vi "AO Reg UI.vi"(8 "error in (no error)":errorcluster, 11 "Node Ptr":T4 format="%.0x") -> (0 "error out":errorcluster)   [LabVIEW 2015, in "Modbus Master System Explorer.lvlib"]
uses:
  Modbus Master System Explorer.lvlib
  <vilib>/NI Veristand/Custom Device API/Custom Device Item Ref.ctl
  Shared/Controls/Data Model/DataType.ctl
  SubVIs/Radix.ctl
  SubVIs/Direction.ctl
  <vilib>/NI VeriStand/Custom Device API/Custom Device API.lvlib
  Shared/Modbus Master Shared.lvlib
panel:
  in  "Direction":T1
  in  "Radix":T2
  out "Bytes":i32
  in  "Sub-Index (Bool)":u16
  in  "DataType":T3
  in  "Valid?":string
  in  "Address":u16
  in  "Header":cluster{"Section Name":string}={"Section Name"="Holding Register (Analog Out) Settings"}
  in  "Description":string
  in  "Name":string
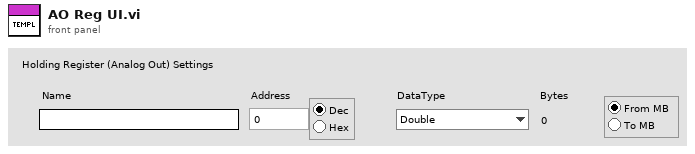
[diagram p1: front panel]
types:
  T1 = typedef "Modbus Master System Explorer.lvlib/Direction.ctl" = enum32{"Radio Selection 1", "Radio Selection 2"}
  T2 = typedef "Modbus Master System Explorer.lvlib/Radix.ctl" = enum32{"Decimal", "Hexidecimal"}
  T3 = typedef "Modbus Master Shared.lvlib/DataType.ctl" = enum16{"Double", "Single", "I64", "I32", "I16", "I8", "U64", "U32", "U16", "U8", "Boolean"}
  T4 = typedef "Custom Device API.lvlib/Custom Device Item Ref.ctl" = u64
  T5 = typedef "Custom Device API.lvlib/Custom Device Item Info.ctl" = cluster{"Name":string, "Is Channel":bool, "GUID":string, "Is Waveform":bool}
  T6 = typedef "Modbus Master Shared.lvlib/Mapping.ctl" = cluster{"DataType":T3, "Starting Address":u16, "Sub-Index (Bool)":u16, "VS Reference":T4}
  T7 = typedef "Custom Device API.lvlib/Custom Device Commands.ctl" = enum16{"Default", "Item renamed", "Shutdown", "Dynamic button pressed"}
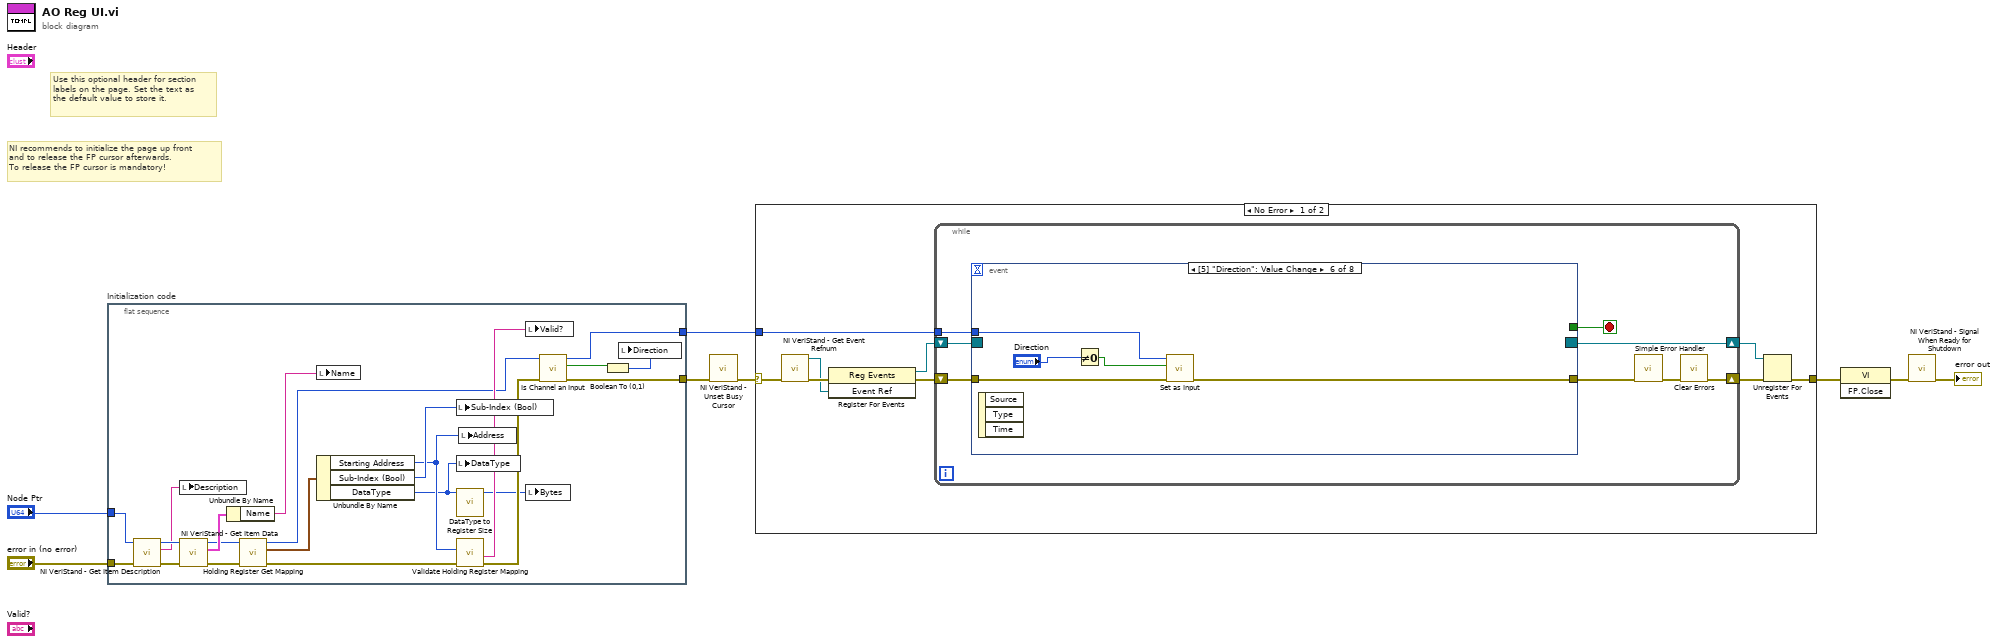
[diagram p0: block diagram]
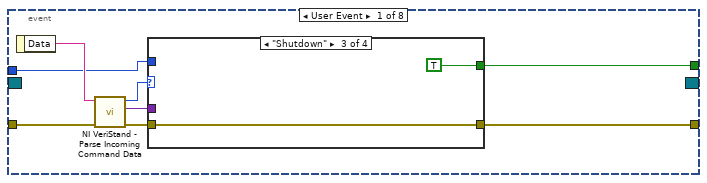
[diagram p2: hidden frame]
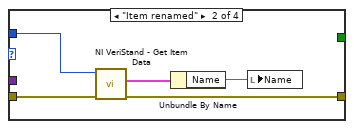
[diagram p4: hidden frame]
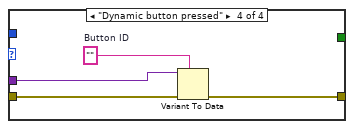
[diagram p5: hidden frame]
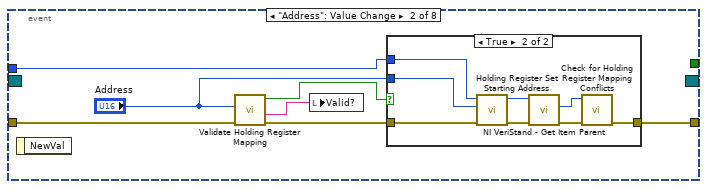
[diagram p6: hidden frame]
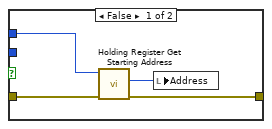
[diagram p7: hidden frame]
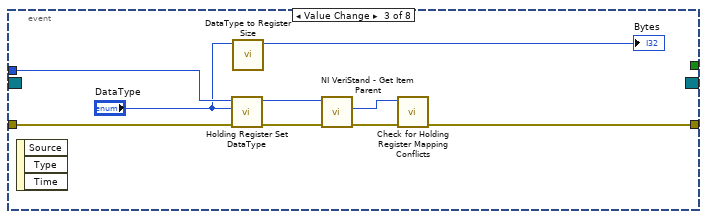
[diagram p8: hidden frame]
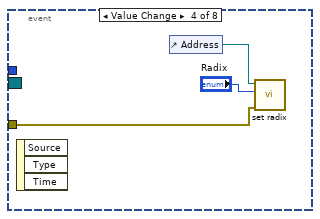
[diagram p9: hidden frame]
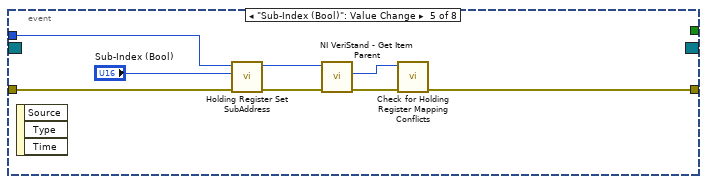
[diagram p10: hidden frame]
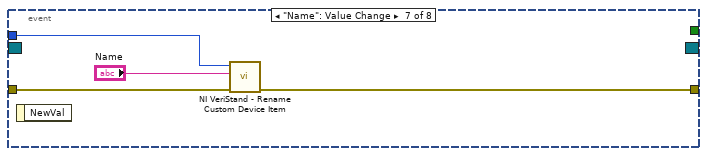
[diagram p11: hidden frame]
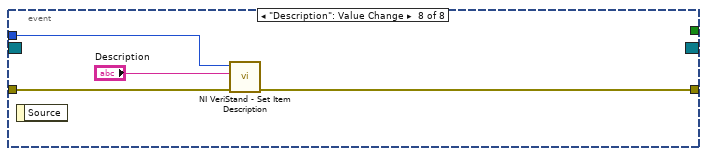
[diagram p12: hidden frame]
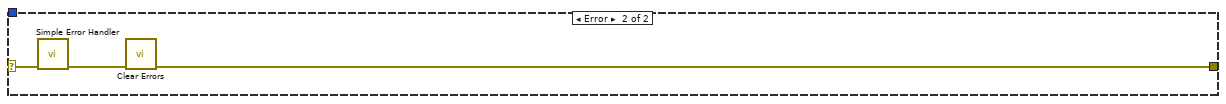
[diagram p13: hidden frame]
diagram:
  # "Use this optional header for section labels on the page. Set the text as the default value to store it."
  # "NI recommends to initialize the page up front\nand to release the FP cursor afterwards.\nTo release the FP cursor is mandatory!"
  n1 = flat-sequence "Initialization code" {
    tunnel: "error in (no error)" -> [w29]
    tunnel: "Node Ptr" -> [w28]
    tunnel: [w20] -> w4
    tunnel: [w22] -> w1
    frame #0 {
      n2 = call <vilib>:"NI VeriStand - Get Item Description.vi"("error in (no error)"=w29, "Item Ref in"=w28) -> ("error out"=w26:errorcluster, "Description"=w27:string, "Item Ref out"=w30:T4)  [unwired: 7 out]
      n3 = local write "Description"(w27) -> ()
      n4 = call <vilib>:"NI VeriStand - Get Item Data.vi"("error in (no error)"=w26, "Item Ref in"=w30) -> ("error out"=w19:errorcluster, "Item Info"=w25:T5, "Item Ref out"=w16:T4)  [unwired: 7 out]
      n5 = Unbundle By Name(w25) -> ("Name"=w24:string)
      n6 = call "Holding Register Get Mapping.vi"("error in (no error)"=w19, "Item Ref in"=w16) -> ("error out"=w18:errorcluster, "Mapping"=w17:T6, "Item Ref out"=w15:T4)  [unwired: 7 in]
      n7 = local write "Name"(w24) -> ()
      n8 = Unbundle By Name(w17) -> ("Starting Address"=w13:u16, "Sub-Index (Bool)"=w14:u16, "DataType"=w11:T3)
      n9 = local write "Sub-Index (Bool)"(w14) -> ()
      n10 = local write "DataType"(w11) -> ()
      n11 = call "DataType to Register Size.vi"("DataType"=w11) -> ("bytes"=w12:i32)  [unwired: 9 in, 1 out]
      n12 = call "Validate Holding Register Mapping.vi"("error in (no error)"=w18, "Mapping"=w13) -> ("error out"=w21:errorcluster, "Status Message"=w23:string)  [unwired: 7 in, 1 out]
      n13 = local write "Address"(w13) -> ()
      n14 = local write "Valid?"(w23) -> ()
      n15 = local write "Bytes"(w12) -> ()
      n16 = call "Is Channel an Input"("error in (no error)"=w21, "Item Ref in"=w15) -> ("error out"=w20:errorcluster, "input?"=w9:bool, "Channel Ref out"=w22:T4)  [unwired: 7 in]
      n17 = Boolean To (0,1)(Boolean=w9) -> (0, 1=w10:i16)
      n18 = local write "Direction"(w10) -> ()
    }
  }
  n19 = call <vilib>:"NI VeriStand - Unset Busy Cursor.vi"("error in (no error)"=w4) -> ("error out"=w3:errorcluster)  [unwired: 10 out]
  n20 = case shown="No Error" w3 {
    selector: w3 -> [w31 w122]
    tunnel: [w36 w120] -> w8
    tunnel: w1 -> [w32 _]
    frame No Error {
      n21 = call <vilib>:"NI VeriStand - Get Event Refnum.vi"("error in (no error)"=w31) -> ("error out"=w39:errorcluster, "Event Ref"=w35:refnum<user-event>)  [unwired: 9 out]
      n22 = register-events(error in=w39, w35) -> (reference out=w33:refnum<event-registration>, error out=w34:errorcluster)  [unwired: 1 in]
      n23 = while {
        tunnel: w32 -> [w43]
        shift-right: [w40] -> w37
        shift-left: w34 -> [w46]
        shift-right: [w47] -> w38
        shift-left: w33 -> [w45]
        stop <- w44 stop-if-true
        n24 = event shown="[5] \"Direction\": Value Change" {
          selector: w45 -> [_ _ _ _ _ _ _ _]
          dyn-events: [_ _ _ _ _ _ _ _] -> w47
          timeout: _ -> [_ _ _ _ _ _ _ _]
          tunnel: w46 -> [w55 w74 w95 w97 w104 w110 w115 w118]
          tunnel: [w51 _ _ _ _ _ _ _] -> w44
          tunnel: [w50 w71 w89 _ w100 w109 w114 w117] -> w42
          tunnel: w43 -> [w49 w73 w94 _ w106 w111 w113 w119]
          event User Event {
            n25 = event-data() -> ("Data"=w54:string)  [unwired: 1 out]
            n26 = call <vilib>:"NI VeriStand - Parse Incoming Command Data.vi"("error in (no error)"=w55, "Incoming data"=w54) -> ("error out"=w53:errorcluster, "Outgoing data"=w48:variant, "Action"=w52:T7)  [unwired: 7 out]
            n27 = case shown="\"Shutdown\"" w52 {
              tunnel: w53 -> [w56 w61 w62 w67]
              tunnel: [_ _ TRUE _] -> w51
              tunnel: [w56 w58 w62 w64] -> w50
              tunnel: w49 -> [_ w60 _ _]
              tunnel: w48 -> [_ _ _ w66]
              frame "Default", Default {
              }
              frame "Item renamed" {
                n28 = call <vilib>:"NI VeriStand - Get Item Data.vi"("error in (no error)"=w61, "Item Ref in"=w60) -> ("error out"=w58:errorcluster, "Item Info"=w59:T5)  [unwired: 8 out]
                n29 = Unbundle By Name(w59) -> ("Name"=w57:string)
                n30 = local write "Name"(w57) -> ()
              }
              frame "Shutdown" {
              }
              frame "Dynamic button pressed" {
                w65 = ""  # Button ID
                n31 = Variant To Data(error in=w67, type=w65, Variant=w66) -> (error out=w64:errorcluster)  [unwired: 1 out]
              }
            }
          }
          event "Address": Value Change {
            n32 = event-data() -> ()  [unwired: 2 out]
            n33 = call "Validate Holding Register Mapping.vi"("error in (no error)"=w74, "Mapping"="Address") -> ("error out"=w72:errorcluster, "Status Message"=w68:string, "Valid?"=w70:bool)  [unwired: 7 in]
            n34 = local write "Valid?"(w68) -> ()
            n35 = case shown="True" w70 {
              tunnel: w73 -> [w78 w85]
              tunnel: w72 -> [w77 w86]
              tunnel: [w76 w79] -> w71
              tunnel: "Address" -> [_ w84]
              frame False {
                n36 = call "Holding Register Get Starting Address.vi"("error in (no error)"=w77, "Item Ref in"=w78) -> ("error out"=w76:errorcluster, "Value"=w75:u16)  [unwired: 7 in, 1 out]
                n37 = local write "Address"(w75) -> ()
              }
              frame True {
                n38 = call "Holding Register Set Starting Address.vi"("error in (no error)"=w86, "Value"=w84, "Item Ref in"=w85) -> ("error out"=w83:errorcluster, "Item Ref out"=w82:T4)  [unwired: 7 in]
                n39 = call <vilib>:"NI VeriStand - Get Item Parent.vi"("error in (no error)"=w83, "Item Ref in"=w82) -> ("error out"=w80:errorcluster, "Parent Ref"=w81:T4)  [unwired: 6 in, 2 out]
                n40 = call "Check for Holding Register Mapping Conflicts.vi"("error in (no error)"=w80, "Group Ref in"=w81) -> ("error out"=w79:errorcluster)  [unwired: 6 in, 3 out]
              }
            }
          }
          event Value Change {
            n41 = event-data() -> ()  [unwired: 4 out]
            n42 = call "Holding Register Set DataType.vi"("error in (no error)"=w95, "DataType"="DataType", "Item Ref in"=w94) -> ("error out"=w90:errorcluster, "Item Ref out"=w92:T4)  [unwired: 7 in]
            n43 = call "DataType to Register Size.vi"("DataType"="DataType") -> ("bytes"=→"Bytes":i32)  [unwired: 9 in, 1 out]
            n44 = call <vilib>:"NI VeriStand - Get Item Parent.vi"("error in (no error)"=w90, "Item Ref in"=w92) -> ("error out"=w91:errorcluster, "Parent Ref"=w93:T4)  [unwired: 6 in, 2 out]
            n45 = call "Check for Holding Register Mapping Conflicts.vi"("error in (no error)"=w91, "Group Ref in"=w93) -> ("error out"=w89:errorcluster)  [unwired: 6 in, 3 out]
          }
          event Value Change {
            n46 = event-data() -> ()  [unwired: 4 out]
            n47 = control-ref of="Address"() -> (w96:refnum<vi>)
            n48 = call "set radix.vi"("error in (no error)"=w97, "Radix"="Radix", "Digital in"=w96) -> ()  [unwired: 8 in, 1 out]
          }
          event "Sub-Index (Bool)": Value Change {
            n49 = event-data() -> ()  [unwired: 4 out]
            n50 = call "Holding Register Set SubAddress.vi"("error in (no error)"=w104, "Value"="Sub-Index (Bool)", "Item Ref in"=w106) -> ("error out"=w102:errorcluster, "Item Ref out"=w99:T4)  [unwired: 7 in]
            n51 = call <vilib>:"NI VeriStand - Get Item Parent.vi"("error in (no error)"=w102, "Item Ref in"=w99) -> ("error out"=w101:errorcluster, "Parent Ref"=w103:T4)  [unwired: 6 in, 2 out]
            n52 = call "Check for Holding Register Mapping Conflicts.vi"("error in (no error)"=w101, "Group Ref in"=w103) -> ("error out"=w100:errorcluster)  [unwired: 6 in, 3 out]
          }
          event Value Change {
            n53 = event-data() -> ()  [unwired: 4 out]
            n54 = Not Equal To 0?(x="Direction") -> (x != 0?=w107:bool)
            n55 = call "Set as Input.vi"("error in (no error)"=w110, "Direction"=w107, "Channel Ref in"=w111) -> ("error out"=w109:errorcluster)  [unwired: 7 in, 1 out]
          }
          event "Name": Value Change {
            n56 = event-data() -> ()  [unwired: 2 out]
            n57 = call <vilib>:"NI VeriStand - Rename Custom Device Item.vi"("error in (no error)"=w115, "New Name"="Name", "Item Ref in"=w113) -> ("error out"=w114:errorcluster)  [unwired: 1 in, 7 out]
          }
          event "Description": Value Change {
            n58 = event-data() -> ()  [unwired: 2 out]
            n59 = call <vilib>:"NI VeriStand - Set Item Description.vi"("error in (no error)"=w118, "Description"="Description", "Item Ref in"=w119) -> ("error out"=w117:errorcluster)  [unwired: 8 out]
          }
        }
        n60 = call <vilib>:"Simple Error Handler.vi"("error in (no error)"=w42) -> ("error out"=w41:errorcluster)  [unwired: 1 in, 7 out]
        n61 = call <vilib>:"Clear Errors.vi"("error in (no error)"=w41) -> ("error out"=w40:errorcluster)  [unwired: 1 in, 5 out]
      }
      n62 = Unregister For Events(event registration refnum=w38, error in=w37) -> (error out=w36:errorcluster)
    }
    frame Error {
      n63 = call <vilib>:"Simple Error Handler.vi"("error in (no error)"=w122) -> ("error out"=w121:errorcluster)  [unwired: 1 in, 7 out]
      n64 = call <vilib>:"Clear Errors.vi"("error in (no error)"=w121) -> ("error out"=w120:errorcluster)  [unwired: 1 in, 5 out]
    }
  }
  n65 = invoke class="VI" method="FP.Close"(error in=w8) -> (error out=w7:errorcluster)  [unwired: 2 in, 2 out]
  n66 = call <vilib>:"NI VeriStand - Signal When Ready for Shutdown.vi"("error in (no error)"=w7) -> ("error out"=→"error out":errorcluster)  [unwired: 10 out]
